vi "CtoFtoK.vi"() -> ()   [LabVIEW 2014]
panel:
  in  "Boolean":bool
  out "kelvin":dbl
  out "celsius":dbl
  out "kelvin":dbl
  out "Fahrenheit":dbl
  in  "Fahrenheit":dbl
  in  "Celsius":dbl
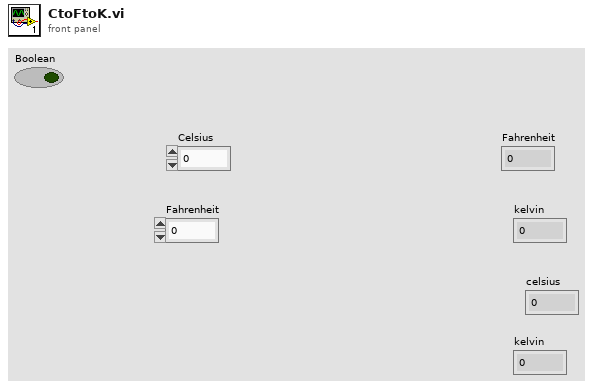
[diagram p1: front panel]
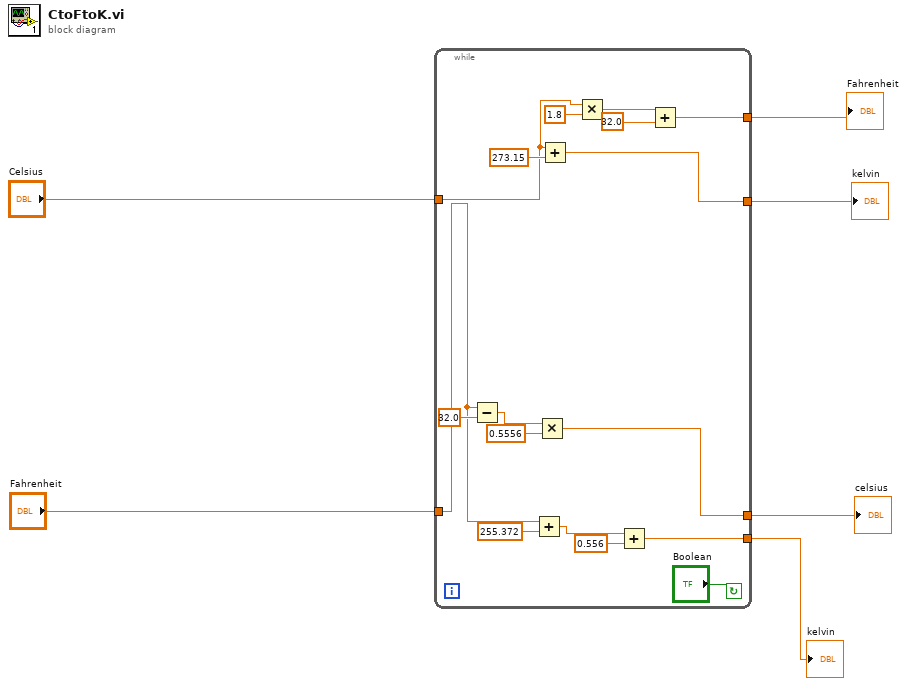
[diagram p0: block diagram]
diagram:
  n1 = while {
    tunnel: [w22] -> w6
    tunnel: "Celsius" -> [w20]
    tunnel: [w17] -> w4
    tunnel: [w15] -> w3
    tunnel: "Fahrenheit" -> [w12]
    tunnel: [w8] -> w1
    stop <- "Boolean" continue-if-true
    n2 = Subtract(x=w12, y=32.0) -> (x-y=w16:dbl)
    n3 = Add(x=w12, y=255.372) -> (x+y=w10:dbl)
    n4 = Multiply(x=w16, y=0.5556) -> (x*y=w15:dbl)
    n5 = Add(x=w20, y=273.15) -> (x+y=w22:dbl)
    n6 = Multiply(x=w20, y=1.8) -> (x*y=w18:dbl)
    n7 = Add(x=w10, y=0.556) -> (x+y=w8:dbl)
    n8 = Add(x=w18, y=32.0) -> (x+y=w17:dbl)
  }
  "Fahrenheit" <- w4
  "kelvin" <- w6
  "celsius" <- w3
  "kelvin" <- w1
